vi "Write Image Information.vi"(8 "error in (no error)":errorcluster, 10 "CCD Config":T1={"Exposure Time"=0.0, "Pre-amp gain"=0, "Readout Rate"=0, "EM Mode"=0, "EM Gain"=2, "Binning"=1, "Initial Line"=1, "Initial Cloumn"=1, "Final Line"=1024, "Final Column"=1024, "Kinetic Series Length"=0, "Shutter Mode"=0, "Cooler ON/OFF"=0, "Temperature"=20, "Current Temperature"=0, "Temperatue Status"="", "Serial Number"=0, "Cubes"=0} {"Temperature" min=0 max=0; "EM Mode" items=["Electron Multiplying", "Conventional"]; "Readout Rate" items=["1 MHz", "10 MHz", "20 MHz", "30 MHz"]; "Pre-amp gain" items=["Gain 1", "Gain 2"]}, 11 "Save Image in":refnum<class "Save Image.lvclass">) -> (0 "error out":errorcluster, 3 "Save Image out":refnum<class "Save Image.lvclass">)   [LabVIEW 2018, in "Save Image.lvclass"]
uses:
  Save Image.lvclass
  Save Image.lvclass/Save Image.ctl
  Simulated_Header/Simulated_Header.lvclass
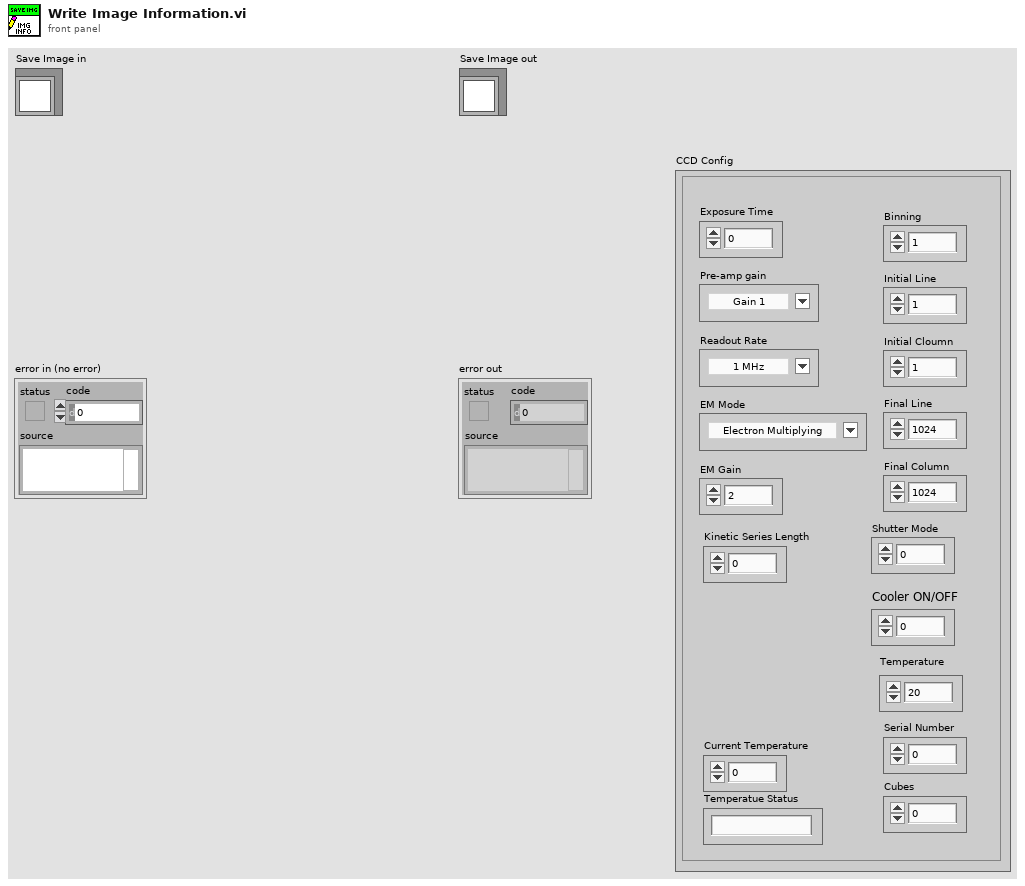
[diagram p1: front panel]
types:
  T1 = cluster{"Exposure Time":sgl, "Pre-amp gain":u8, "Readout Rate":u8, "EM Mode":u8, "EM Gain":u16, "Binning":u16, "Initial Line":u16, "Initial Cloumn":u16, "Final Line":u16, "Final Column":u16, "Kinetic Series Length":u32, "Shutter Mode":u8, "Cooler ON/OFF":u8, "Temperature":i8, "Current Temperature":i16, "Temperatue Status":string, "Serial Number":u16, "Cubes":u32}
  T2 = cluster{"FILENAME":cluster{"Name":string, "Value":string, "Comment":string}, "OBSERVER":cluster{"Name":string, "Value":string, "Comment":string}, "PROGRID":cluster{"Name":string, "Value":string, "Comment":string}, "OBJECT":cluster{"Name":string, "Value":string, "Comment":string}, "NIGHTDIR":cluster{"Name":string, "Value":string, "Comment":string}, "CHANNEL":cluster{"Name":string, "Value":string, "Comment":string}, "INSTRUME":cluster{"Name":string, "Value":string, "Comment":string}, "NEXPSEQ":cluster{"Name":string, "Value":string, "Comment":string}, "SEQINDEX":cluster{"Name":string, "Value":string, "Comment":string}, "OBSTYPE":cluster{"Name":string, "Value":string, "Comment":string}, "READMOD":cluster{"Name":string, "Value":string, "Comment":string}, "READMODE":cluster{"Name":string, "Value":string, "Comment":string}, "ACQMODE":cluster{"Name":string, "Value":string, "Comment":string}, "PREAMP":cluster{"Name":string, "Value":string, "Comment":string}, "READOUT":cluster{"Name":string, "Value":string, "Comment":string}, "VSHIFT":cluster{"Name":string, "Value":string, "Comment":string}, "TRIGGER":cluster{"Name":string, "Value":string, "Comment":string}, "EMMODE":cluster{"Name":string, "Value":string, "Comment":string}, "EMGAIN":cluster{"Name":string, "Value":string, "Comment":string}, "VBIN":cluster{"Name":string, "Value":string, "Comment":string}, "HBIN":cluster{"Name":string, "Value":string, "Comment":string}, "INITLIN":cluster{"Name":string, "Value":string, "Comment":string}, "INITCOL":cluster{"Name":string, "Value":string, "Comment":string}, "FINALLIN":cluster{"Name":string, "Value":string, "Comment":string}, "FINALCOL":cluster{"Name":string, "Value":string, "Comment":string}, "KSERLEN":cluster{"Name":string, "Value":string, "Comment":string}, "SHUTTER":cluster{"Name":string, "Value":string, "Comment":string}, "OPENSHT":cluster{"Name":string, "Value":string, "Comment":string}, "CLOSESHT":cluster{"Name":string, "Value":string, "Comment":string}, "DATE":cluster{"Name":string, "Value":string, "Comment":string}, "GAIN":cluster{"Name":string, "Value":string, "Comment":string}, "GAINERR":cluster{"Name":string, "Value":string, "Comment":string}, "RDNOISE":cluster{"Name":string, "Value":string, "Comment":string}, "RNOISERR":cluster{"Name":string, "Value":string, "Comment":string}, "SKYFIBER":cluster{"Name":string, "Value":string, "Comment":string}, "CALFIBER":cluster{"Name":string, "Value":string, "Comment":string}, "UTDATE":cluster{"Name":string, "Value":string, "Comment":string}, "LOCTIME":cluster{"Name":string, "Value":string, "Comment":string}, "MJD":cluster{"Name":string, "Value":string, "Comment":string}, "OBSLON":cluster{"Name":string, "Value":string, "Comment":string}, "OBSLAT":cluster{"Name":string, "Value":string, "Comment":string}, "OBSALT":cluster{"Name":string, "Value":string, "Comment":string}, "EXPTIME":cluster{"Name":string, "Value":string, "Comment":string}, "TELRA":cluster{"Name":string, "Value":string, "Comment":string}, "TELDEC":cluster{"Name":string, "Value":string, "Comment":string}, "RA":cluster{"Name":string, "Value":string, "Comment":string}, "DEC":cluster{"Name":string, "Value":string, "Comment":string}, "RA_DEG":cluster{"Name":string, "Value":string, "Comment":string}, "DEC_DEG":cluster{"Name":string, "Value":string, "Comment":string}, "EPOCH":cluster{"Name":string, "Value":string, "Comment":string}, "HA":cluster{"Name":string, "Value":string, "Comment":string}, "HAD":cluster{"Name":string, "Value":string, "Comment":string}, "AIRMASS":cluster{"Name":string, "Value":string, "Comment":string}, "AMSTART":cluster{"Name":string, "Value":string, "Comment":string}, "AMEND":cluster{"Name":string, "Value":string, "Comment":string}, "XOFFSET":cluster{"Name":string, "Value":string, "Comment":string}, "YOFFSET":cluster{"Name":string, "Value":string, "Comment":string}, "PA":cluster{"Name":string, "Value":string, "Comment":string}, "CAMFOC":cluster{"Name":string, "Value":string, "Comment":string}, "TELFOC":cluster{"Name":string, "Value":string, "Comment":string}, "TCSUT":cluster{"Name":string, "Value":string, "Comment":string}, "TCSST":cluster{"Name":string, "Value":string, "Comment":string}, "MOONDIST":cluster{"Name":string, "Value":string, "Comment":string}, "MOONALT":cluster{"Name":string, "Value":string, "Comment":string}, "MOONPHAS":cluster{"Name":string, "Value":string, "Comment":string}, "ADC":cluster{"Name":string, "Value":string, "Comment":string}, "ADCSPEED":cluster{"Name":string, "Value":string, "Comment":string}, "CALMIRR":cluster{"Name":string, "Value":string, "Comment":string}, "GUIDING":cluster{"Name":string, "Value":string, "Comment":string}, "GUIDTEXP":cluster{"Name":string, "Value":string, "Comment":string}, "GUIDFREQ":cluster{"Name":string, "Value":string, "Comment":string}, "GUIDOBJX":cluster{"Name":string, "Value":string, "Comment":string}, "GUIDOBJY":cluster{"Name":string, "Value":string, "Comment":string}, "AVGYCORR":cluster{"Name":string, "Value":string, "Comment":string}, "AVGXCORR":cluster{"Name":string, "Value":string, "Comment":string}, "GFOCUS":cluster{"Name":string, "Value":string, "Comment":string}, "THARLAMP":cluster{"Name":string, "Value":string, "Comment":string}, "HALLAMP":cluster{"Name":string, "Value":string, "Comment":string}, "AGITATOR":cluster{"Name":string, "Value":string, "Comment":string}, "THARMIRR":cluster{"Name":string, "Value":string, "Comment":string}, "DSTATUS":cluster{"Name":string, "Value":string, "Comment":string}, "DPOS":cluster{"Name":string, "Value":string, "Comment":string}, "DTEMP":cluster{"Name":string, "Value":string, "Comment":string}, "DHUM":cluster{"Name":string, "Value":string, "Comment":string}, "DLAMP":cluster{"Name":string, "Value":string, "Comment":string}, "DFLAT":cluster{"Name":string, "Value":string, "Comment":string}, "TEMPEXT":cluster{"Name":string, "Value":string, "Comment":string}, "PRESSURE":cluster{"Name":string, "Value":string, "Comment":string}, "HUMIDITY":cluster{"Name":string, "Value":string, "Comment":string}, "WINDDIR":cluster{"Name":string, "Value":string, "Comment":string}, "WINSPEED":cluster{"Name":string, "Value":string, "Comment":string}, "SHTTTL":cluster{"Name":string, "Value":string, "Comment":string}, "COOLER":cluster{"Name":string, "Value":string, "Comment":string}, "TEMP":cluster{"Name":string, "Value":string, "Comment":string}, "TEMPST":cluster{"Name":string, "Value":string, "Comment":string}, "SERN":cluster{"Name":string, "Value":string, "Comment":string}, "OBS_TITLE":cluster{"Name":string, "Value":string, "Comment":string}, "COMMENT":cluster{"Name":string, "Value":string, "Comment":string}, "SIMPLE":cluster{"Name":string, "Value":string, "Comment":string}, "NAXIS":cluster{"Name":string, "Value":string, "Comment":string}, "EXTEND":cluster{"Name":string, "Value":string, "Comment":string}}
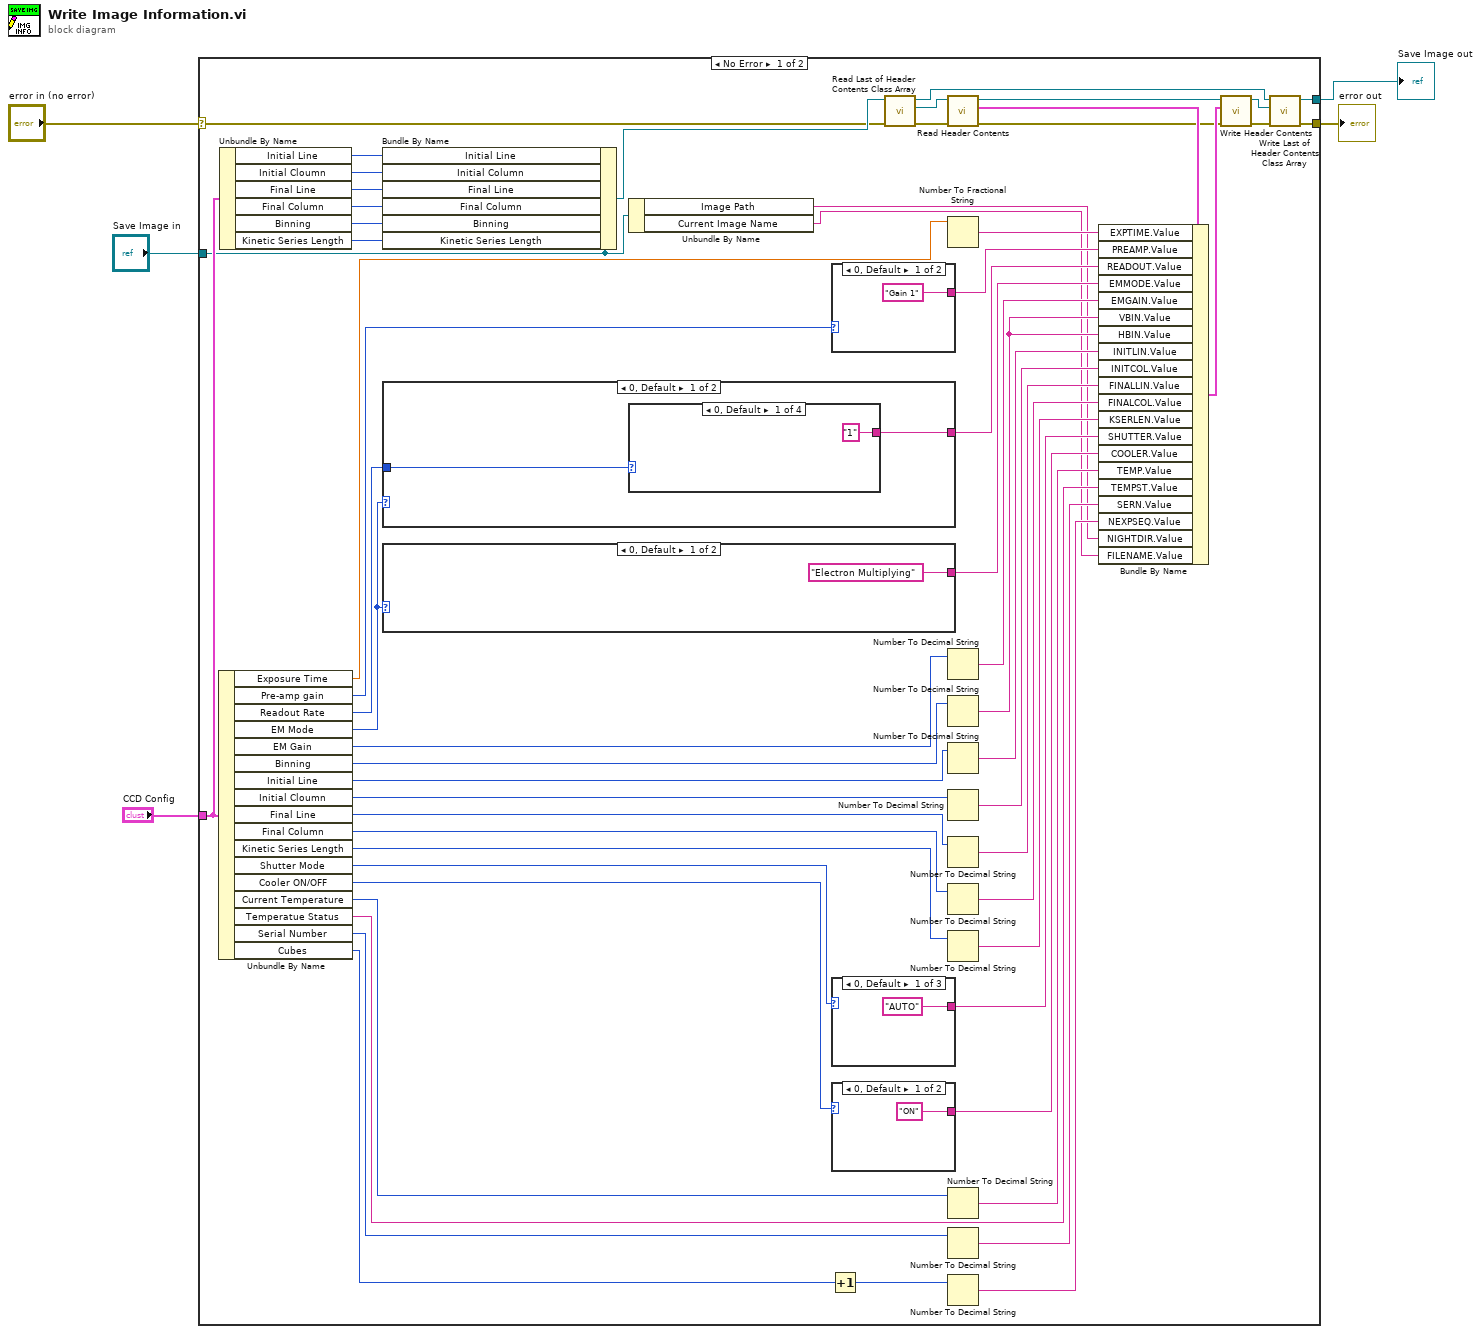
[diagram p0: block diagram]
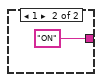
[diagram p2: hidden frame]
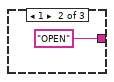
[diagram p3: hidden frame]
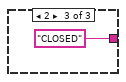
[diagram p4: hidden frame]
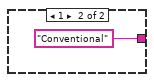
[diagram p5: hidden frame]
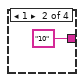
[diagram p6: hidden frame]
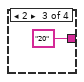
[diagram p7: hidden frame]
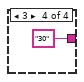
[diagram p8: hidden frame]
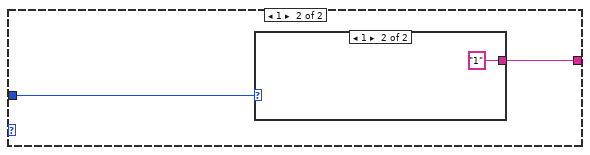
[diagram p9: hidden frame]
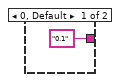
[diagram p10: hidden frame]
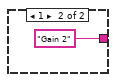
[diagram p11: hidden frame]
diagram:
  n1 = case shown="No Error" "error in (no error)" {
    selector: "error in (no error)" -> [w20 w82]
    tunnel: [w19 w82] -> w4
    tunnel: [w18 w83] -> w2
    tunnel: "Save Image in" -> [w8 w83]
    tunnel: "CCD Config" -> [w56 _]
    frame No Error {
      n2 = Unbundle By Name(w56) -> ("Exposure Time"=w55:sgl, "Pre-amp gain"=w54:u8, "Readout Rate"=w53:u8, "EM Mode"=w52:u8, "EM Gain"=w51:u16, "Binning"=w50:u16, "Initial Line"=w49:u16, "Initial Cloumn"=w48:u16, "Final Line"=w47:u16, "Final Column"=w46:u16, "Kinetic Series Length"=w45:u32, "Shutter Mode"=w44:u8, "Cooler ON/OFF"=w43:u8, "Current Temperature"=w42:i16, "Temperatue Status"=w24:string, "Serial Number"=w41:u16, "Cubes"=w39:u32)
      n3 = Unbundle By Name(w56) -> ("Initial Line"=w62:u16, "Initial Cloumn"=w61:u16, "Final Line"=w60:u16, "Final Column"=w59:u16, "Binning"=w58:u16, "Kinetic Series Length"=w57:u32)
      n4 = Bundle By Name(cluster=w8, "Initial Line"=w62, "Initial Column"=w61, "Final Line"=w60, "Final Column"=w59, "Binning"=w58, "Kinetic Series Length"=w57) -> (w21:refnum<class "Save Image.lvclass">)
      n5 = case shown="0, Default" w52 {
        tunnel: w53 -> [w71 w77]
        tunnel: [w70 w76] -> w36
        frame 0, Default {
          n6 = case shown="0, Default" w71 {
            tunnel: ["1" "10" "20" "30"] -> w70
            frame 0, Default {
            }
            frame 1 {
            }
            frame 2 {
            }
            frame 3 {
            }
          }
        }
        frame 1 {
          n7 = case shown="1" w77 {
            tunnel: ["0.1" "1"] -> w76
            frame 0, Default {
            }
            frame 1 {
            }
          }
        }
      }
      n8 = case shown="0, Default" w52 {
        tunnel: ["Electron Multiplying" "Conventional"] -> w35
        frame 0, Default {
        }
        frame 1 {
        }
      }
      n9 = Unbundle By Name(w8) -> ("Image Path"=w7:string, "Current Image Name"=w6:string)
      n10 = Increment(x=w39) -> (x+1=w40:u32)
      n11 = case shown="0, Default" w54 {
        tunnel: ["Gain 1" "Gain 2"] -> w37
        frame 0, Default {
        }
        frame 1 {
        }
      }
      n12 = case shown="0, Default" w44 {
        tunnel: ["AUTO" "OPEN" "CLOSED"] -> w27
        frame 0, Default {
        }
        frame 1 {
        }
        frame 2 {
        }
      }
      n13 = case shown="0, Default" w43 {
        tunnel: ["ON" "ON"] -> w26
        frame 0, Default {
        }
        frame 1 {
        }
      }
      n14 = call "Read Last of Header Contents Class Array.vi"("error in (no error)"=w20, "Save Image in"=w21) -> ("error out"=w11:errorcluster, "Simulated_Header.lvclass"=w12:refnum<class "Simulated_Header.lvclass">, "Save Image out"=w9:refnum<class "Save Image.lvclass">)  [unwired: 7 in]
      n15 = call "Read Header Contents.vi"("error in (no error)"=w11, "Header in"=w12) -> ("error out"=w10:errorcluster, "Header Content"=w16:T2, "Header out"=w15:refnum<class "Simulated_Header.lvclass">)  [unwired: 7 in]
      n16 = Number To Fractional String(number=w55) -> (F-format string=w38:string)  [unwired: 3 in]
      n17 = Number To Decimal String(number=w51) -> (decimal integer string=w34:string)  [unwired: 1 in]
      n18 = Number To Decimal String(number=w50) -> (decimal integer string=w33:string)  [unwired: 1 in]
      n19 = Number To Decimal String(number=w49) -> (decimal integer string=w32:string)  [unwired: 1 in]
      n20 = Number To Decimal String(number=w48) -> (decimal integer string=w31:string)  [unwired: 1 in]
      n21 = Number To Decimal String(number=w47) -> (decimal integer string=w30:string)  [unwired: 1 in]
      n22 = Number To Decimal String(number=w46) -> (decimal integer string=w29:string)  [unwired: 1 in]
      n23 = Number To Decimal String(number=w45) -> (decimal integer string=w28:string)  [unwired: 1 in]
      n24 = Number To Decimal String(number=w42) -> (decimal integer string=w25:string)  [unwired: 1 in]
      n25 = Number To Decimal String(number=w41) -> (decimal integer string=w23:string)  [unwired: 1 in]
      n26 = Number To Decimal String(number=w40) -> (decimal integer string=w22:string)  [unwired: 1 in]
      n27 = Bundle By Name(cluster=w16, "EXPTIME.Value"=w38, "PREAMP.Value"=w37, "READOUT.Value"=w36, "EMMODE.Value"=w35, "EMGAIN.Value"=w34, "VBIN.Value"=w33, "HBIN.Value"=w33, "INITLIN.Value"=w32, "INITCOL.Value"=w31, "FINALLIN.Value"=w30, "FINALCOL.Value"=w29, "KSERLEN.Value"=w28, "SHUTTER.Value"=w27, "COOLER.Value"=w26, "TEMP.Value"=w25, "TEMPST.Value"=w24, "SERN.Value"=w23, "NEXPSEQ.Value"=w22, "NIGHTDIR.Value"=w7, "FILENAME.Value"=w6) -> (w17:T2)
      n28 = call "Write Header Contents.vi"("error in (no error)"=w10, "Header Content"=w17, "Header in"=w15) -> ("error out"=w13:errorcluster, "Header out"=w14:refnum<class "Simulated_Header.lvclass">)  [unwired: 7 in]
      n29 = call "Write Last of Header Contents Class Array.vi"("error in (no error)"=w13, "Simulated_Header.lvclass"=w14, "Save Image in"=w9) -> ("error out"=w19:errorcluster, "Save Image out"=w18:refnum<class "Save Image.lvclass">)  [unwired: 7 in]
    }
    frame Error {
    }
  }
  "error out" <- w4
  "Save Image out" <- w2
